vi "Generate Class HTML Documentation.vi"(4 "Root Folder Name":string="Toolkit", 6 "Requirement":string="Labstache", 7 "Destination":path=path "", 8 "Error In":errorcluster, 11 "Class File":path=path "") -> (0 "Error Out":errorcluster)   [LabVIEW 2018, in "Scripts.lvlib"]
uses:
  Scripts.lvlib
  Toolkit/Data/Map/Map.lvclass
  D:/Users/cfield/Code/Field R&D Services/Mustache/LabVIEW/trunk/src/Toolkit/Data/Datum/Datum.lvclass
  Toolkit/Data/Array/Array.lvclass
  Toolkit/Data/Pair/Support/From String.vi
  Toolkit/Data/Array/Support/From Data.vi
  Toolkit/Data/Pair/Support/From Datum.vi
  Toolkit/Data/Map/Support/From Pair Array.vi
  Toolkit/Data/Pair/Pair.lvclass
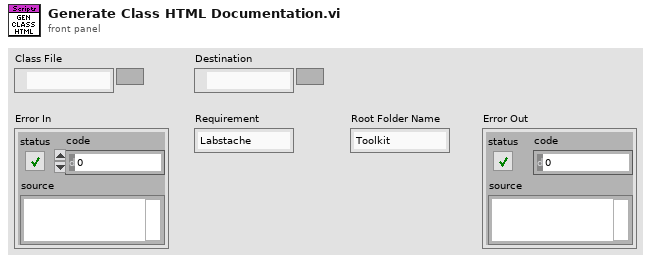
[diagram p1: front panel]
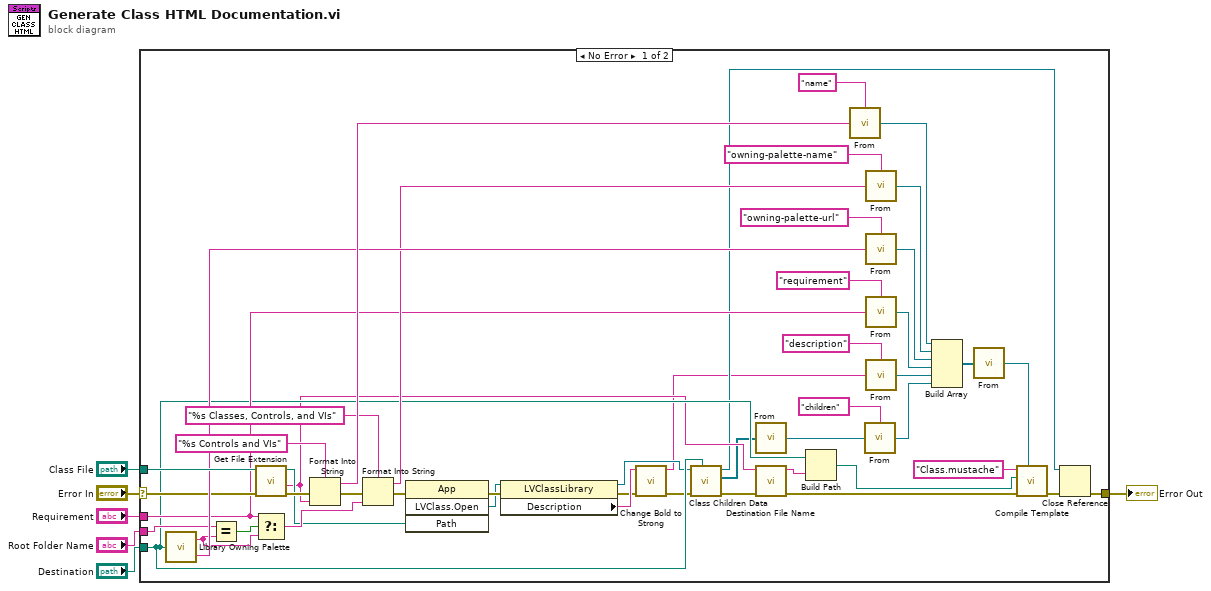
[diagram p0: block diagram]
diagram:
  n1 = case shown="No Error" "Error In" {
    selector: "Error In" -> [w43 w56]
    tunnel: "Destination" -> [w36 _]
    tunnel: "Class File" -> [w55 _]
    tunnel: [w45 w56] -> w5
    tunnel: "Root Folder Name" -> [w41 _]
    tunnel: "Requirement" -> [w37 _]
    frame No Error {
      n2 = call "Library Owning Palette.vi"("Destination"=w36) -> ("Name"=w38:string, "URL"=w51:string)
      n3 = Equal?(x=w41, y=w38) -> (x = y?=w39:bool)
      n4 = call <vilib>:"Get File Extension.vi"("error in (no error)"=w43, "file"=w55) -> ("error out"=w48:errorcluster, "filename without extension"=w35:string, "dup file"=w46:path)  [unwired: 5 in, 2 out]
      n5 = Select(t=w37, s=w39, f=w38) -> (s? t:f=w47:string)
      n6 = Format Into String(format string="%s Controls and VIs", error in=w48, w35) -> (resulting string=w54:string, error out=w52:errorcluster)  [unwired: 1 in]
      n7 = Format Into String(format string="%s Classes, Controls, and VIs", error in=w52, w47) -> (resulting string=w50:string, error out=w49:errorcluster)  [unwired: 1 in]
      n8 = invoke class="App" method="LVClass.Open"(error in=w49, "Path"=w46) -> (error out=w44:errorcluster, "LVClass.Open"=w42:refnum<vi>)  [unwired: 2 in, 2 out]
      n9 = property class="LVClassLibrary"(reference=w42, error in=w44) -> (reference out=w33:refnum<vi>, error out=w32:errorcluster, "Description"=w40:string)
      n10 = call "Change Bold to Strong.vi"("Error In"=w32, "Bold Description"=w40) -> ("Error Out"=w9:errorcluster, "Strong Description"=w10:string)  [unwired: 8 in]
      n11 = call "Class Children Data.vi"("Destination"=w36, "Error In"=w9, "Class In"=w33) -> ("Error Out"=w15:errorcluster, "Array"=w14:refnum<class "Map.lvclass">[], "Class Out"=w16:refnum<vi>)  [unwired: 6 in]
      n12 = call-poly "From.vi"("Data"=w14) -> ("Array"=w13:refnum<class "Array.lvclass">)  [unwired: 1 in]
      n13 = call "Destination File Name.vi"("Error In"=w15, "File Stem"=w35) -> ("Error Out"=w21:errorcluster, "Destination File Name"=w22:string)  [unwired: 8 in]
      n14 = Build Path(base path=w36, name or relative path=w22) -> (appended path=w23:path)
      n15 = call-poly "From.vi"("Value"=w54, "Key"="name") -> ("Pair"=w27:refnum<class "Pair.lvclass">)
      n16 = call-poly "From.vi"("Value"=w13, "Key"="children") -> ("Pair"=w11:refnum<class "Pair.lvclass">)
      n17 = call-poly "From.vi"("Value"=w50, "Key"="owning-palette-name") -> ("Pair"=w28:refnum<class "Pair.lvclass">)
      n18 = call-poly "From.vi"("Value"=w51, "Key"="owning-palette-url") -> ("Pair"=w29:refnum<class "Pair.lvclass">)
      n19 = call-poly "From.vi"("Value"=w37, "Key"="requirement") -> ("Pair"=w7:refnum<class "Pair.lvclass">)
      n20 = call-poly "From.vi"("Value"=w10, "Key"="description") -> ("Pair"=w17:refnum<class "Pair.lvclass">)
      n21 = Build Array(w27, w28, w29, w7, w17, w11) -> (w30:refnum<class "Pair.lvclass">[])
      n22 = call-poly "From.vi"("Pairs"=w30) -> ("Map"=w31:refnum<class "Map.lvclass">)  [unwired: 1 in]
      n23 = call "Compile Template.vi"("Data"=w31, "Error In"=w21, "Output"=w23, "Template File Name"="Class.mustache" ("name or relative path")) -> ("Error Out"=w20:errorcluster)  [unwired: 7 in]
      n24 = Close Reference(reference=w16, error in (no error)=w20) -> (error out=w45:errorcluster)
    }
    frame Error {
    }
  }
  "Error Out" <- w5
